vi "SetResume.vi"(8 "error in":errorcluster, 11 "VISA resource name":refnum<visa-resource-name>) -> (0 "error out":errorcluster, 2 "Resume result":string, 3 "VISA resource name out":refnum<visa-resource-name>)   [LabVIEW 2023, in "Thermotron 8800.lvlib"]
doc: "RESM\nCommand name: Resume program or manual mode operation\nCommand type: Control\nDescription: Returns a program or test from hold mode to its run mode.\nSyntax: RESM\nData type: No data\nQuery example: RESM\n8800 response: The program or test returns to run mode."
uses:
  Thermotron 8800.lvlib
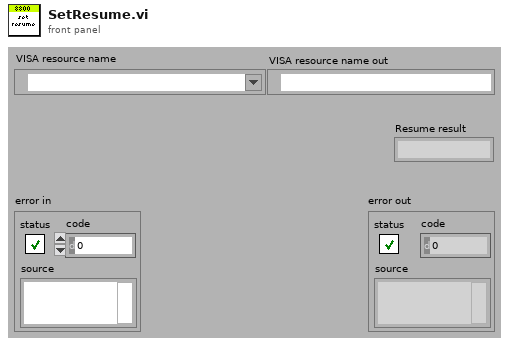
[diagram p1: front panel]
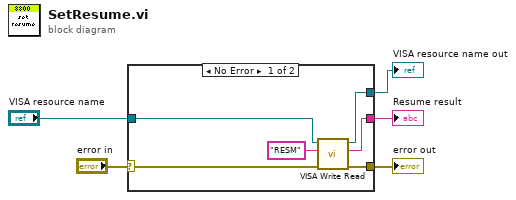
[diagram p0: block diagram]
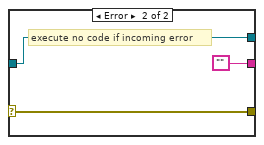
[diagram p2: hidden frame]
diagram:
  n1 = case shown="No Error" "error in" {
    selector: "error in" -> [w7 w14]
    tunnel: "VISA resource name" -> [w10 w13]
    tunnel: [w9 w13] -> w4
    tunnel: [w8 w14] -> w3
    tunnel: [w6 ""] -> w1
    frame No Error {
      n2 = call "VISA Write Read.vi"("error in (no error)"=w7, "8800 Command"="RESM", "VISA Refnum in"=w10) -> ("error out"=w8:errorcluster, "read buffer"=w6:string, "VISA Refnum out"=w9:refnum<visa-resource-name>)  [unwired: 6 in]
    }
    frame Error {
      # "execute no code if incoming error"
    }
  }
  "VISA resource name out" <- w4
  "error out" <- w3
  "Resume result" <- w1
